vi "FWHM&Profiles.vi"(0 "image array":dbl[][](array[numeric]) format="%.2f") -> (1 "x max index":i32, 2 "y max index":i32, 3 "Xprofile":dbl[](array[numeric]) format="%.2f", 4 "FWHMX":dbl format="%.2f", 5 "Yprofile":dbl[](array[numeric]) format="%.2f", 6 "FWHMY":dbl format="%.2f")   [LabVIEW 2011]
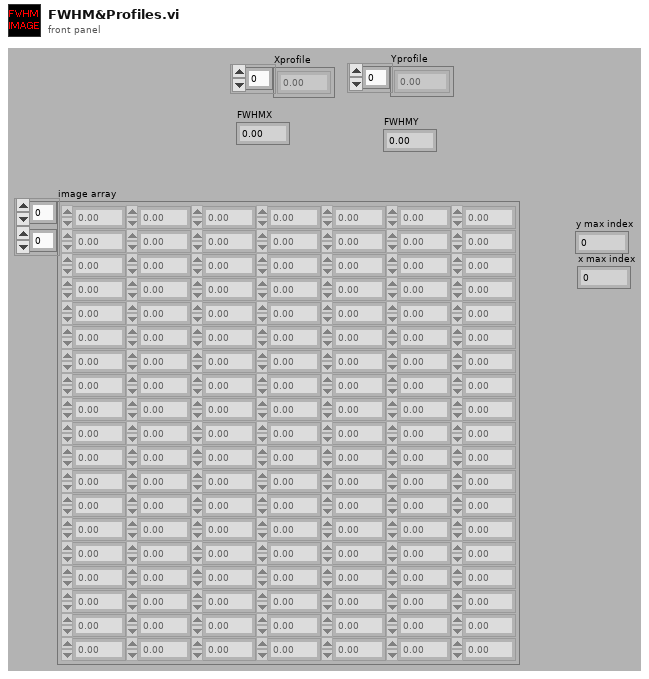
[diagram p1: front panel]
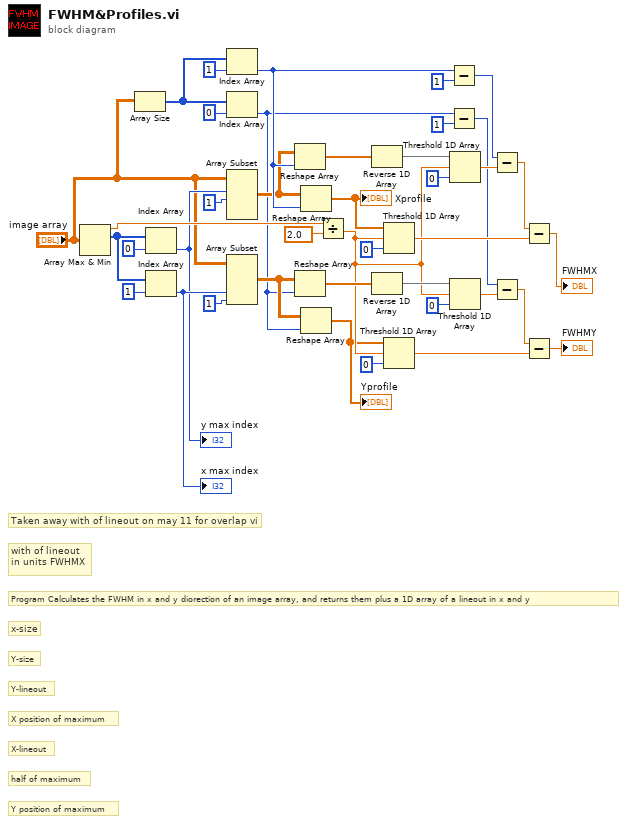
[diagram p0: block diagram]
diagram:
  # "Taken away with of lineout on may 11 for overlap vi"
  # "with of lineout in units FWHMX"
  # "Program Calculates the FWHM in x and y diorection of an image array, and returns them plus a 1D array of a lineout in x and y"
  # "x-size"
  # "Y-size"
  # "Y-lineout"
  # "X position of maximum"
  # "X-lineout"
  # "half of maximum"
  # "Y position of maximum"
  n1 = Array Max & Min(array="image array") -> (max value=w38:dbl, max index (indices)=w33:i32[])  [unwired: 2 out]
  n2 = Array Size(array="image array") -> (size(s)=w28:i32[])
  n3 = Index Array(array=w33, index=0) -> (element=w4:i32)
  "y max index" <- w4
  n4 = Index Array(array=w33, index=1) -> (element=w7:i32)
  "x max index" <- w7
  n5 = Index Array(array=w28, index=1) -> (element=w40:i32)
  n6 = Index Array(array=w28, index=0) -> (element=w8:i32)
  n7 = Array Subset(array="image array", index (row)=w4, length (row)=1 ("length")) -> (w39:dbl[][])  [unwired: 2 in]
  n8 = Array Subset(array="image array", index (col)=w7, length (col)=1 ("length")) -> (w10:dbl[][])  [unwired: 2 in]
  n9 = Reshape Array(w39, w40) -> (w27:dbl[])
  n10 = Reshape Array(w10, w8) -> (w18:dbl[])
  n11 = Reshape Array(w39, w40) -> (w3:dbl[])
  "Xprofile" <- w3
  n12 = Reshape Array(w10, w8) -> (w1:dbl[])
  "Yprofile" <- w1
  n13 = Divide(x=w38, y=2.0) -> (x/y=w9:dbl)
  n14 = Reverse 1D Array(array=w27) -> (reversed array=w26:dbl[])
  n15 = Reverse 1D Array(array=w18) -> (reversed array=w17:dbl[])
  n16 = Threshold 1D Array(1:0 ("start index (0)"), 2:w9, 3:w3) -> (0:w20:dbl)
  n17 = Threshold 1D Array(1:0 ("start index (0)"), 2:w9, 3:w1) -> (0:w11:dbl)
  n18 = Subtract(x=w40, y=1) -> (x-y=w22:i32)
  n19 = Subtract(x=w8, y=1) -> (x-y=w13:i32)
  n20 = Threshold 1D Array(1:0 ("start index (0)"), 2:w9, 3:w26) -> (0:w24:dbl)
  n21 = Threshold 1D Array(1:0 ("start index (0)"), 2:w9, 3:w17) -> (0:w15:dbl)
  n22 = Subtract(x=w22, y=w24) -> (x-y=w21:dbl)
  n23 = Subtract(x=w13, y=w15) -> (x-y=w12:dbl)
  n24 = Subtract(x=w21, y=w20) -> (x-y=→"FWHMX":dbl)
  n25 = Subtract(x=w12, y=w11) -> (x-y=→"FWHMY":dbl)
